vi "Get Platform Path Separator.vi"() -> (0 "platform path separator":string)   [LabVIEW 2013, in "VITesterUtilities.lvlib"]
doc: "Returns the path separator for the platform on which the software is running, as shown below:\n\nWindows: \"\\\" (backslash)\nLinux: \"/\" (slash)\nMac: \":\" (colon)"
uses:
  Libraries/VITesterUtilities.lvlib
panel:
  # "Copyright © 2007 James Kring, Inc. All rights reserved.\n\nAuthor: Jim Kring <jim.kring@jameskring.com>\n\nThis library is provided \"AS IS\" , WITHOUT WARRANTIES OR \nCONDITIONS OF ANY KIND, either express or implied.\n\nJames Kring, Inc. -- http://www.jameskring.com"
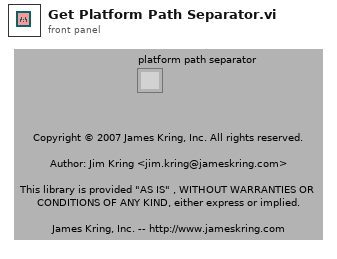
[diagram p1: front panel]
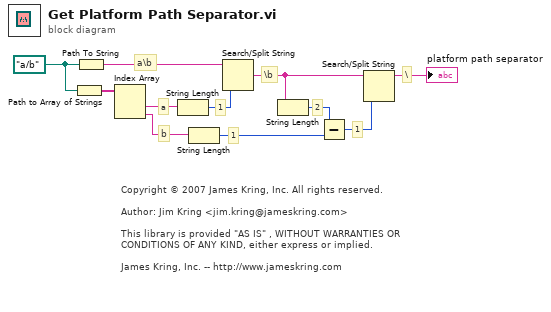
[diagram p0: block diagram]
diagram:
  w11 = path "a/b"
  # "Copyright © 2007 James Kring, Inc. All rights reserved.\n\nAuthor: Jim Kring <jim.kring@jameskring.com>\n\nThis library is provided \"AS IS\" , WITHOUT WARRANTIES OR \nCONDITIONS OF ANY KIND, either express or implied.\n\nJames Kring, Inc. -- http://www.jameskring.com"
  # "1"
  # "2"
  # "1"
  # "1"
  # "\\"
  # "\\b"
  # "b"
  # "a"
  # "a\\b"
  n1 = Path to Array of Strings(0:w11) -> (2:w10:string[])  [unwired: 1 out]
  n2 = Path To String(path=w11) -> (string=w7:string)
  n3 = Index Array(array=w10) -> (element #1=w9:string, element #2=w8:string)  [unwired: 2 in]
  n4 = String Length(string=w9) -> (length=w6:i32)
  n5 = String Length(string=w8) -> (length=w4:i32)
  n6 = Search/Split String(string=w7, offset (0)=w6) -> (match + rest of string=w1:string)  [unwired: 1 in, 2 out]
  n7 = String Length(string=w1) -> (length=w5:i32)
  n8 = Subtract(x=w5, y=w4) -> (x-y=w3:i32)
  n9 = Search/Split String(string=w1, offset (0)=w3) -> (substring before match=→"platform path separator":string)  [unwired: 1 in, 2 out]
